vi "FPGA_driver.vi"() -> ()   [LabVIEW 2019]
uses:
  <vilib>/Platform/TimedLoop/XDataNode/timing_clust.ctl
  <vilib>/Platform/TimedLoop/XDataNode/nitl_modes.ctl
  <vilib>/Platform/TimedLoop/XDataNode/wakeup.ctl
  <vilib>/rvi/Emulation/niFpgaGetClockAttributes.vi
  <vilib>/rvi/Emulation/niFpgaSctlEmulationGetInTimedLoop.vi
  <vilib>/rvi/Emulation/niFpgaEmulationReportErrorSimple.vi
  <vilib>/rvi/Emulation/niFpgaProcessEmulError.vi
  <vilib>/rvi/Emulation/niFpgaCriticalErrorInLSC.vi
  <vilib>/rvi/eio/common/nirviEmuTemplateMethod_errors.vi
  <vilib>/rvi/Analysis/common/FxpNativeNode/niFpgaFxpNative.xnode
  <vilib>/eio/EIONode/EIONode.xnode
  <vilib>/platform/TimedLoop/XDataNode/XDataNode.xnode
  <vilib>/Platform/TimedLoop/XDataNode/XDNodeRunTimeDep.lvlib
panel:
  in  "Coil Current Direction 2":bool
  out "ConnectorC/AO1":i16
  out "ConnectorC/AO0":i16
  in  "ConnectorC/DIO1":bool
  in  "Num_cycle_on":u32
  in  "enable?":bool
  out "Encoder Position 2":i16
  in  "Encoder Reset 2":bool
  in  "Encoder Reload Value 2":i16
  out "clk/pulse":i32
  out "Velocity\nValid?":bool
  in  "Position Ref.":i32
  in  "Num Clocks\nper Period":u32=400000
  in  "Velocity \nLimit":i32=10
  in  "Position Loop\nPeriod (ms)":u32=10
  out "Encoder Position":i16
  in  "Encoder Reset":bool
  in  "Encoder Reload Value":i16
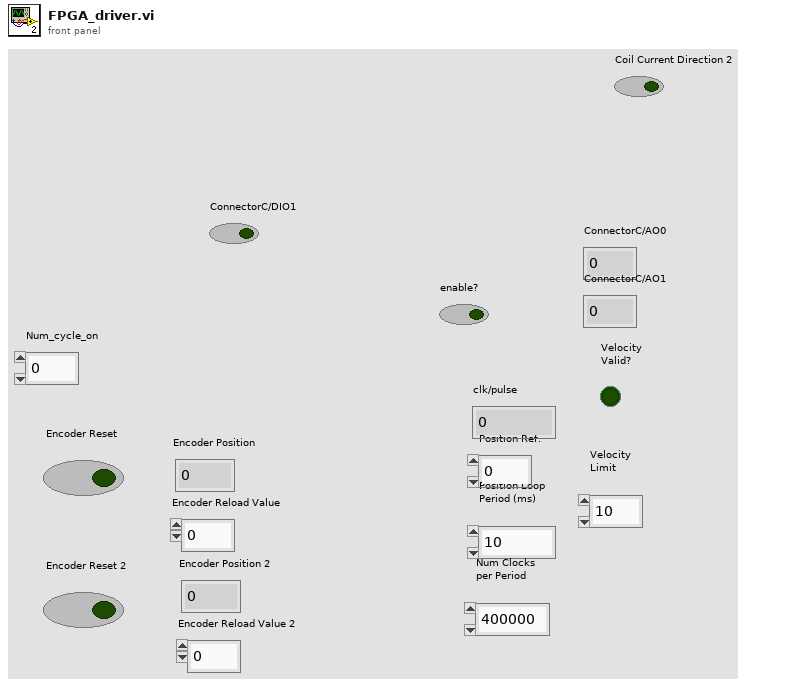
[diagram p1: front panel]
types:
  T1 = typedef "XDNodeRunTimeDep.lvlib/timing_clust.ctl" = cluster{"Expected End [f-1]":u64, "Actual End [f-1]":u64, "Finished Late? [f-1]":bool, "Expected End [i-1]":u64, "Actual End [i-1]":u64, "Finished Late? [i-1]":bool, "Expected Start [i]":u64, "Actual Start [i]":u64, "Expected Start [f]":u64, "Actual Start [f]":u64, "Source Name":string, "Structure Name":string, "Period":i64, "Deadline":i64, "Offset":i64, "Start":i64, "Priority":i32, "Timeout":i32, "Mode":T2, "Wakeup Reason":T3, "Error":errorcluster, "Source Type":string, "Secondary Source Type":string, "Global End Time":u64, "Global Start Time":u64, "Frame Duration":u64, "Iteration Duration":u64, "Assigned CPU":i32, "I/O Scan Engine Mode":u32}
  T2 = typedef "XDNodeRunTimeDep.lvlib/nitl_modes.ctl" = enum32{"No Change", "Process missed periods, maintain original phase", "Discard missed periods, maintain original phase", "Process missed periods, ignore original phase", "Discard missed periods, ignore original phase"}
  T3 = typedef "XDNodeRunTimeDep.lvlib/wakeup.ctl" = enum32{"Normal", "Aborted", "Asynchronous wakeup", "Timing source error", "Timed loop error", "Timeout"}
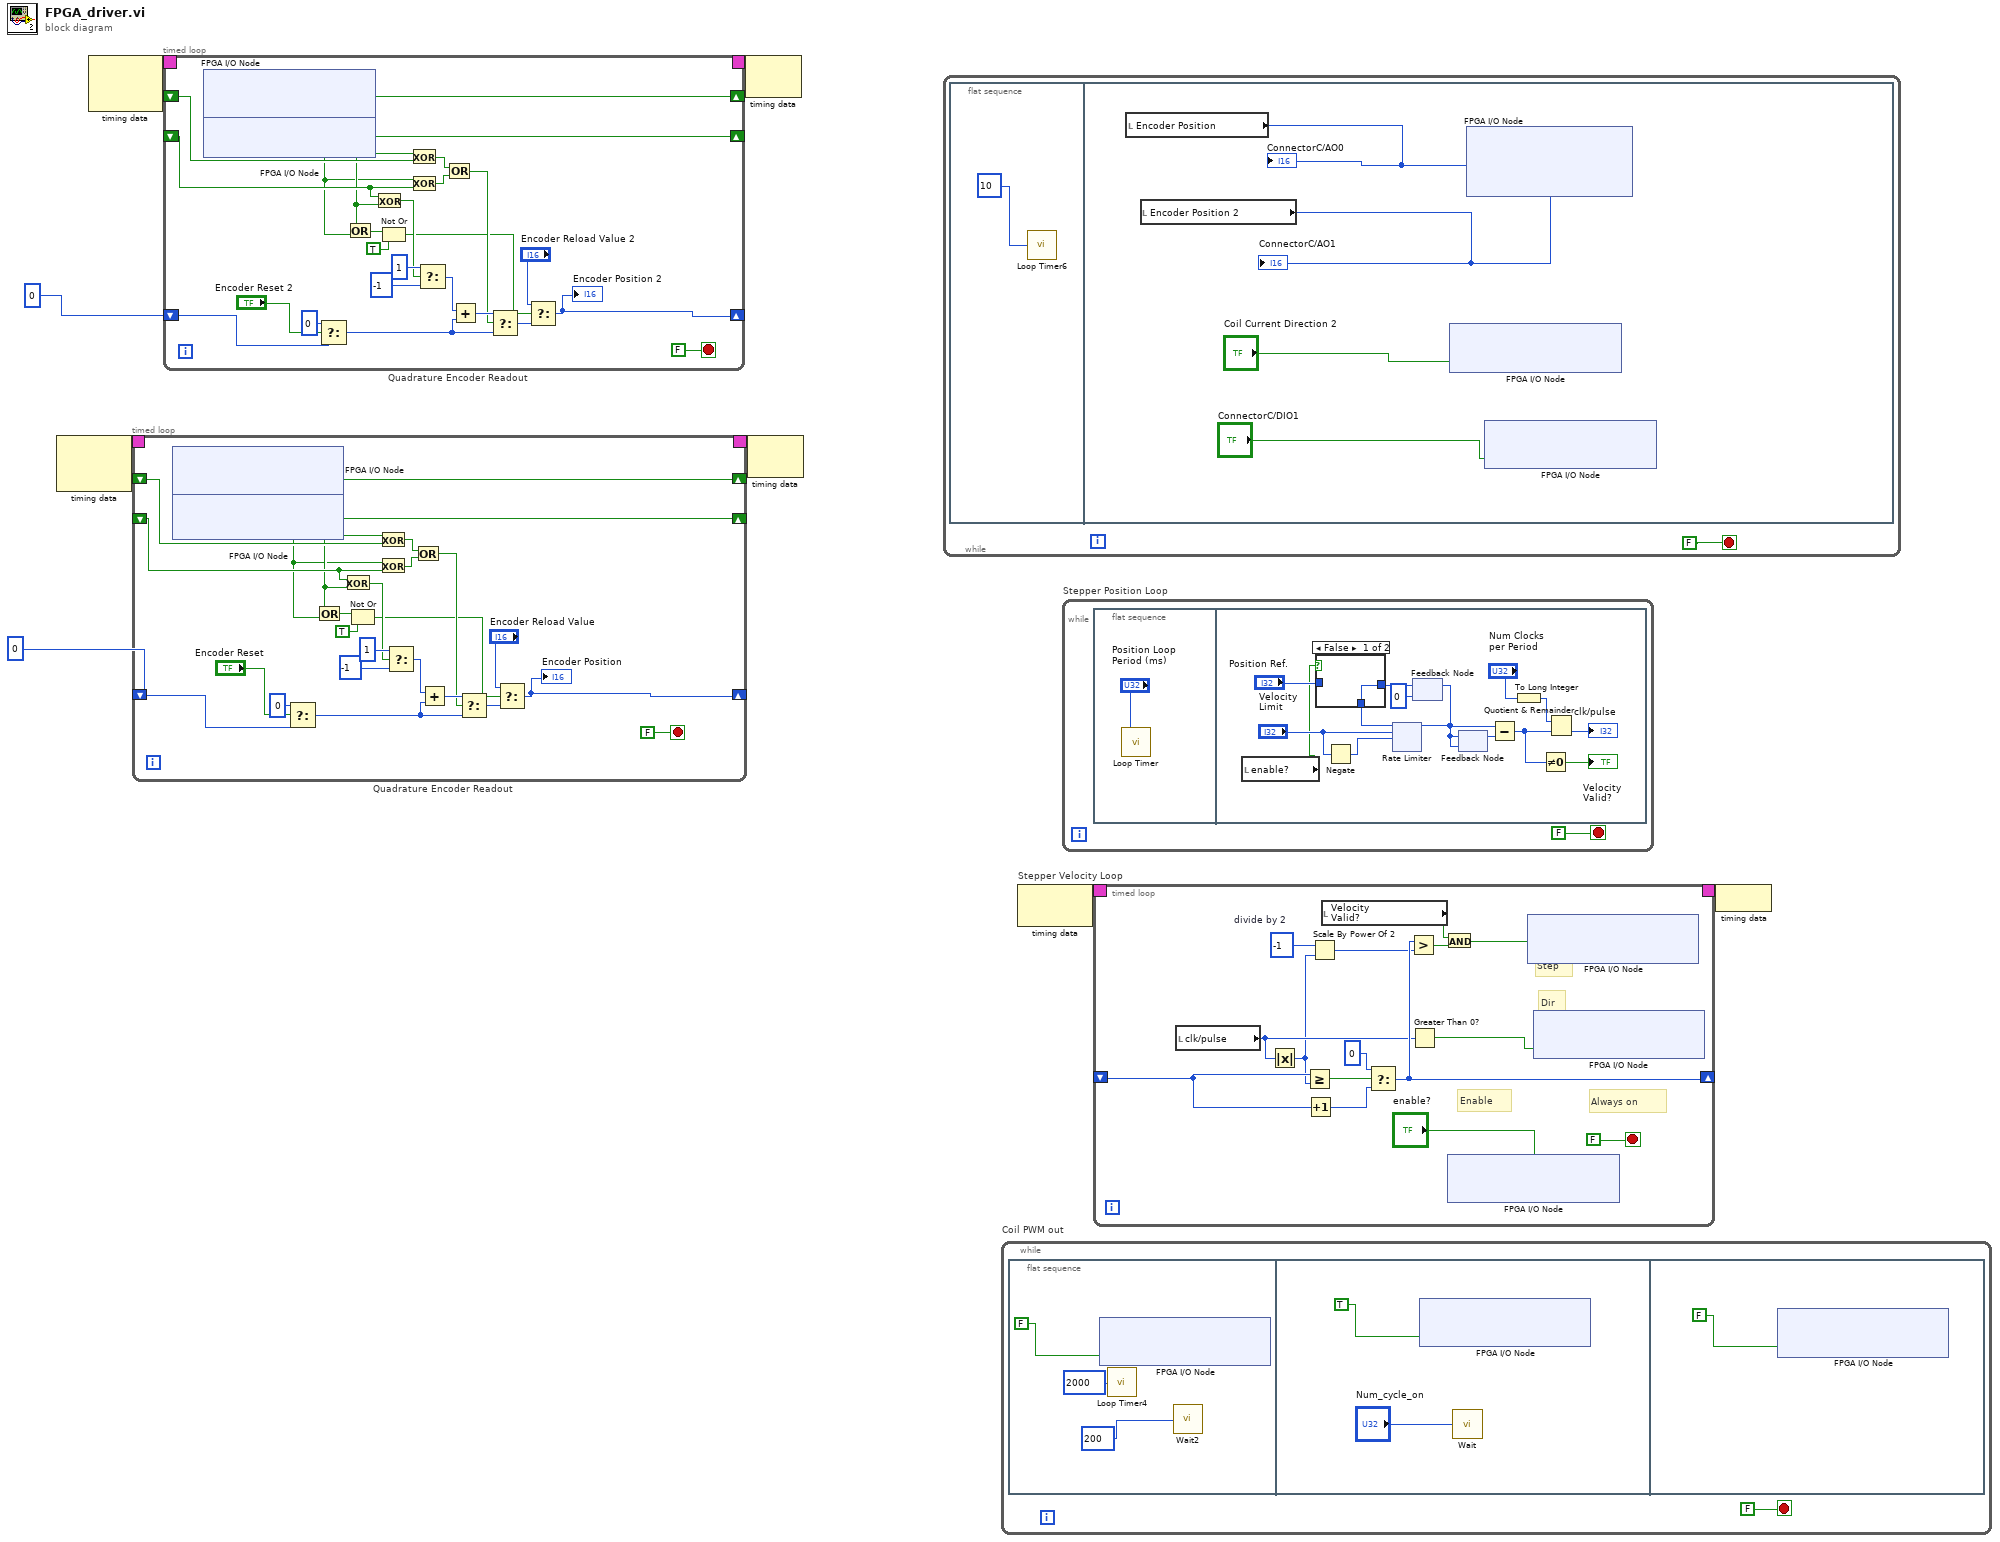
[diagram p0: block diagram]
diagram:
  n1 = node-c288() -> (w8:T1)  [unwired: 2 out]
  n2 = node-c288() -> (w3:T1)  [unwired: 2 out]
  n3 = timed-loop "Quadrature Encoder Readout" {
    timing-out: [_] -> w7
    timing: w8 -> [_]
    shift-left: _ -> [w16]
    shift-right: [w12] -> _
    shift-left: i16 0 -> [w27]
    shift-right: [w9] -> _
    shift-left: _ -> [w17]
    shift-right: [w13] -> _
    stop <- FALSE stop-if-true
    n4 = xnode "FPGA I/O Node"() -> ("ConnectorA/DIO0"=w13:bool)  [unwired: 2 in, 2 out]
    n5 = xnode "FPGA I/O Node"() -> ("ConnectorA/DIO1"=w12:bool)  [unwired: 1 in, 1 out]
    n6 = Select(t=i16 0, s="Encoder Reset", f=w27) -> (s? t:f=w29:i16)
    n7 = Or(x=w13, y=w12) -> (x .or. y?=w11:bool)
    n8 = Exclusive Or(1:w13, 2:w16) -> (0:w18:bool)
    n9 = Not Or(1:TRUE ("y"), 2:w11) -> (0:w15:bool)
    n10 = Exclusive Or(1:w17, 2:w13) -> (0:w20:bool)
    n11 = Exclusive Or(1:w16, 2:w12) -> (0:w21:bool)
    n12 = Select(t=i16 1, s=w18, f=i16 -1) -> (s? t:f=w26:i16)
    n13 = Or(x=w20, y=w21) -> (x .or. y?=w19:bool)
    n14 = Add(x=w26, y=w29) -> (x+y=w31:i16)
    n15 = Select(t=w31, s=w19, f=w29) -> (s? t:f=w23:i16)
    n16 = Select(t="Encoder Reload Value", s=w15, f=w23) -> (s? t:f=w9:i16)
    "Encoder Position" <- w9
  }
  n17 = timed-loop "Quadrature Encoder Readout" {
    timing-out: [_] -> w2
    timing: w3 -> [_]
    shift-left: _ -> [w41]
    shift-right: [w37] -> _
    shift-left: i16 0 -> [w52]
    shift-right: [w34] -> _
    shift-left: _ -> [w42]
    shift-right: [w38] -> _
    stop <- FALSE stop-if-true
    n18 = xnode "FPGA I/O Node"() -> ("ConnectorA/DIO2"=w38:bool)  [unwired: 1 in, 1 out]
    n19 = xnode "FPGA I/O Node"() -> ("ConnectorA/DIO3"=w37:bool)  [unwired: 1 in, 1 out]
    n20 = Select(t=i16 0, s="Encoder Reset 2", f=w52) -> (s? t:f=w54:i16)
    n21 = Or(x=w38, y=w37) -> (x .or. y?=w36:bool)
    n22 = Exclusive Or(1:w38, 2:w41) -> (0:w43:bool)
    n23 = Not Or(1:TRUE ("y"), 2:w36) -> (0:w40:bool)
    n24 = Exclusive Or(1:w42, 2:w38) -> (0:w45:bool)
    n25 = Exclusive Or(1:w41, 2:w37) -> (0:w46:bool)
    n26 = Select(t=i16 1, s=w43, f=i16 -1) -> (s? t:f=w51:i16)
    n27 = Or(x=w45, y=w46) -> (x .or. y?=w44:bool)
    n28 = Add(x=w51, y=w54) -> (x+y=w56:i16)
    n29 = Select(t=w56, s=w44, f=w54) -> (s? t:f=w48:i16)
    n30 = Select(t="Encoder Reload Value 2", s=w40, f=w48) -> (s? t:f=w34:i16)
    "Encoder Position 2" <- w34
  }
  n31 = node-c288(w2) -> ()  [unwired: 1 out]
  n32 = node-c288(w7) -> ()  [unwired: 1 out]
  n33 = while {
    stop <- FALSE stop-if-true
    n34 = flat-sequence {
      frame #0 {
        n35 = call "Loop Timer6"("Count(mSec)"=u32 10) -> ()  [unwired: 1 out]
      }
      frame #1 {
        n36 = local read "Encoder Position"() -> (w62:i16)
        "ConnectorC/AO0" <- w62
        n37 = local read "Encoder Position 2"() -> (w63:i16)
        "ConnectorC/AO1" <- w63
        n38 = xnode "FPGA I/O Node"("ConnectorC/DIO0"="Coil Current Direction 2") -> ()  [unwired: 1 in, 1 out]
        n39 = xnode "FPGA I/O Node"("ConnectorC/AO0"=w62, "ConnectorC/AO1"=w63) -> ()  [unwired: 2 in, 2 out]
        n40 = xnode "FPGA I/O Node"("ConnectorC/DIO1"="ConnectorC/DIO1") -> ()  [unwired: 1 in, 1 out]
      }
    }
  }
  n41 = while "Coil PWM out" {
    stop <- FALSE stop-if-true
    n42 = flat-sequence {
      frame #0 {
        n43 = xnode "FPGA I/O Node"("ConnectorC/DIO1"=FALSE) -> ()  [unwired: 1 in, 1 out]
        n44 = call "Loop Timer4"("Count(Ticks)"=u32 2000 ("Count(uSec)")) -> ()  [unwired: 1 out]
        n45 = call "Wait2"("Count(Ticks)"=u32 200) -> ()  [unwired: 1 out]
      }
      frame #1 {
        n46 = xnode "FPGA I/O Node"("ConnectorC/DIO1"=TRUE) -> ()  [unwired: 1 in, 1 out]
        n47 = call "Wait"("Count(Ticks)"="Num_cycle_on") -> ()  [unwired: 1 out]
      }
      frame #2 {
        n48 = xnode "FPGA I/O Node"("ConnectorC/DIO1"=FALSE) -> ()  [unwired: 1 in, 1 out]
      }
    }
  }
  n49 = node-c288() -> (w5:T1)  [unwired: 1 in]
  n50 = while "Stepper Position Loop" {
    stop <- FALSE stop-if-true
    n51 = flat-sequence {
      frame #0 {
        n52 = call "Loop Timer"("Count(mSec)"="Position Loop\nPeriod (ms)") -> ()  [unwired: 1 out]
      }
      frame #1 {
        n53 = local read "enable?"() -> (w74:bool)
        n54 = Negate(x="Velocity \nLimit") -> (-x=w81:i32)
        n55 = feedback #1(0 ("output")) -> (w76:i32)
        n56 = case shown="False" w74 {
          tunnel: [w88 w89] -> w79
          tunnel: "Position Ref." -> [_ w89]
          tunnel: w76 -> [w88 _]
          frame False {
          }
          frame True {
          }
        }
        n57 = xnode ("Rate Limiter")("pos slew rate * dt"="Velocity \nLimit", "input"=w79, "neg slew rate * dt"=w81) -> ("output"=w77:i32)  [unwired: 1 in]
        n58 = feedback-in #1(w77) -> ()
        n59 = feedback #2(w77) -> (w86:i32)
        n60 = feedback-in #2(w77) -> ()
        n61 = Subtract(x=w77, y=w86) -> (x-y=w83:i32)
        n62 = To Long Integer(number="Num Clocks\nper Period") -> (32bit integer=w84:i32)
        n63 = Not Equal To 0?(x=w83) -> (x != 0?=→"Velocity\nValid?":bool)
        n64 = Quotient & Remainder(x=w84, y=w83) -> (floor(x/y)=→"clk/pulse":i32)  [unwired: 1 out]
      }
    }
  }
  n65 = timed-loop "Stepper Velocity Loop" {
    timing: w5 -> [_]
    timing-out: [_] -> w4
    shift-right: [w124] -> _
    shift-left: _ -> [w121]
    stop <- FALSE stop-if-true
    w117 = -1  # divide by 2
    # "Always on"
    # "Enable"
    # "Dir"
    # "Step"
    n66 = local read "clk/pulse"() -> (w120:i32)
    n67 = Absolute Value(x=w120) -> (abs(x)=w118:i32)
    n68 = Greater Or Equal?(x=w121, y=w118) -> (x >= y?=w125:bool)
    n69 = Increment(x=w121) -> (x+1=w127:i32)
    n70 = Scale By Power Of 2(n=w117, x=w118) -> (x*2^n=w119:i32)
    n71 = local read "Velocity\nValid?"() -> (w122:bool)
    n72 = Select(t=0, s=w125, f=w127) -> (s? t:f=w124:i32)
    n73 = Greater?(x=w124, y=w119) -> (0:w123:bool)
    n74 = Greater Than 0?(x=w120) -> (x > 0?=w116:bool)
    n75 = And(x=w122, y=w123) -> (x .and. y?=w115:bool)
    n76 = xnode "FPGA I/O Node"("ConnectorC/DIO4"="enable?") -> ()  [unwired: 1 in, 1 out]
    n77 = xnode "FPGA I/O Node"("ConnectorC/DIO2"=w115) -> ()  [unwired: 1 in, 1 out]
    n78 = xnode "FPGA I/O Node"("ConnectorC/DIO3"=w116) -> ()  [unwired: 1 in, 1 out]
  }
  n79 = node-c288(w4) -> ()
